vi "Get List of Orphaned Pointers by ID.vi"(6 "Recurse Up List":bool, 7 "Linked List ID":string, 8 "error in (no error)":errorcluster, 10 "Removed Unique ID":string, 11 "Linked List Ref":refnum<data-value>) -> (0 "error out":errorcluster, 2 "Orphaned Pointer IDs":string[](array[string]), 3 "Linked List Ref out":refnum<data-value>)   [LabVIEW 2020, in "Linked Lists.lvlib" / "Linked List Ref.lvclass"]
uses:
  <vilib>/gpm_packages/@cs/linked-list/Source/Linked List/Linked List Ref/Linked List Ref.lvclass
  <vilib>/gpm_packages/@cs/linked-list/Source/Linked List/ILinkedList/ILinked List.lvclass
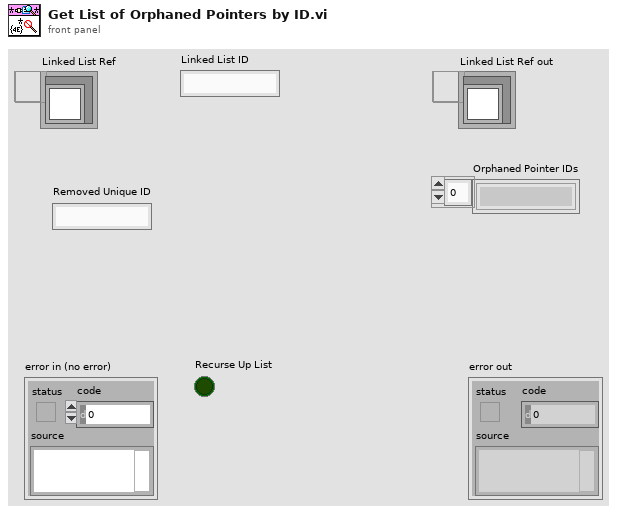
[diagram p1: front panel]
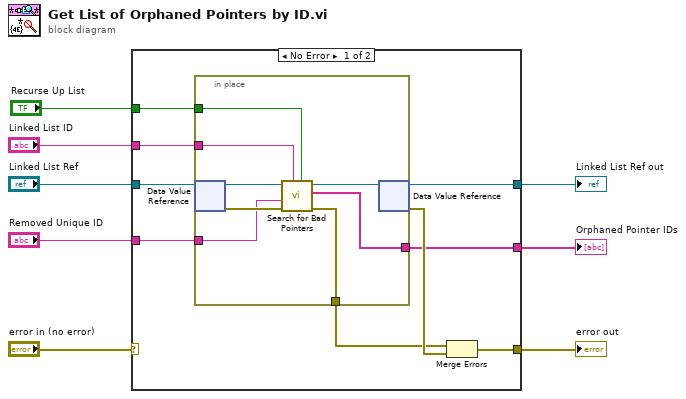
[diagram p0: block diagram]
diagram:
  n1 = case shown="No Error" "error in (no error)" {
    selector: "error in (no error)" -> [_ w27]
    tunnel: "Linked List Ref" -> [w17 w26]
    tunnel: "Linked List ID" -> [w16 _]
    tunnel: [w14 w27] -> w5
    tunnel: [w15 w26] -> w4
    tunnel: "Recurse Up List" -> [w11 _]
    tunnel: "Removed Unique ID" -> [w10 _]
    tunnel: [w9 _] -> w1
    frame No Error {
      n2 = in-place {
        in-place-border: w16 -> [w21]
        in-place-border: [w22] -> w12
        in-place-border: w11 -> [w20]
        in-place-border: w10 -> [w19]
        in-place-border: [w18] -> w9
        n3 = in-place-dvr #1(w17) -> (w25:refnum<class "ILinked List.lvclass">, w23:errorcluster)
        n4 = call-dynamic "Search for Bad Pointers.vi"("Recurse Up List"=w20, "Linked List ID"=w21, "error in (no error)"=w23, "Removed Unique ID"=w19, "ILinked List in"=w25) -> ("error out"=w22:errorcluster, "IDs"=w18:string[], "ILinked List out"=w24:refnum<class "ILinked List.lvclass">)  [unwired: 4 in]
        n5 = in-place-dvr #1(w24) -> (w15:refnum<data-value>, w13:errorcluster)
      }
      n6 = Merge Errors(w12, w13) -> (w14:errorcluster)
    }
    frame Error {
    }
  }
  "error out" <- w5
  "Linked List Ref out" <- w4
  "Orphaned Pointer IDs" <- w1
